vi "Obtain Request Events.vi"(8 "error in":errorcluster, 10 "Create New? (F)":bool) -> (0 "error out":errorcluster, 2 "UI Module Template Request Events":T1)   [LabVIEW 2024, in "UI Module Template.lvlib"]
doc: "This VI Obtains/Creates the Requests events that will be used for other modules to communicate with the module that owns this VI. These Requests events will be accessed only via Public API methods for this module.\n\n<b>NOTE</b>: The contents of this VI are automatically generated and modified by the <b>Tools > DQMH Consortium > DQMH</b> utilities. Consider using those utilities instead of making your own modifications to this VI.\n_____\nBased on DQMH Project Template 7.0.1.1316."
uses:
  UI Module Template.lvlib
  Request Events--cluster.ctl
  Stop Argument--cluster.ctl
  Show Panel Argument--cluster.ctl
  Hide Panel Argument--cluster.ctl
  Get Module Execution Status Argument--cluster.ctl
  Show Diagram Argument--cluster.ctl
  Get UI Reference Argument--cluster.ctl
  Get UI Reference (Reply Payload)--cluster.ctl
  Inserted Into Subpanel Argument--cluster.ctl
  Set Config (String) Argument--cluster.ctl
  Set Config Argument--cluster.ctl
  Config.ctl
  Get config Argument--cluster.ctl
  Get config (Reply Payload)--cluster.ctl
  Get Config (String) Argument--cluster.ctl
  Get Config (String) (Reply Payload)--cluster.ctl
  Generate Dummy Data Argument--cluster.ctl
panel:
  # "NOTE: The contents of this VI are automatically generated and modified by the Tools > DQMH Consortium > DQMH utilities. Consider using those utilities instead of making your own modifications to this VI."
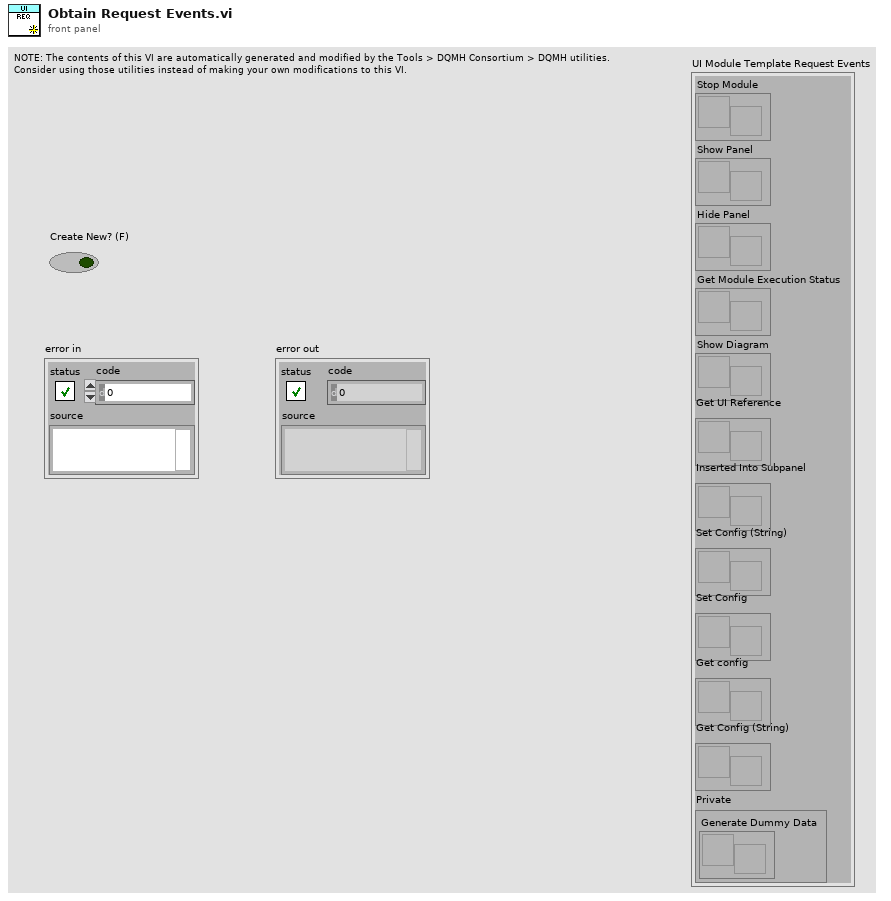
[diagram p1: front panel]
types:
  T1 = typedef "UI Module Template.lvlib/Request Events--cluster.ctl" = cluster{"Stop Module":refnum<user-event>, "Show Panel":refnum<user-event>, "Hide Panel":refnum<user-event>, "Get Module Execution Status":refnum<user-event>, "Show Diagram":refnum<user-event>, "Get UI Reference":refnum<user-event>, "Inserted Into Subpanel":refnum<user-event>, "Set Config (String)":refnum<user-event>, "Set Config":refnum<user-event>, "Get config":refnum<user-event>, "Get Config (String)":refnum<user-event>, "Private":cluster{"Generate Dummy Data":refnum<user-event>}}
  T2 = typedef "UI Module Template.lvlib/Generate Dummy Data Argument--cluster.ctl" = cluster{"Boolean":bool}
  T3 = typedef "UI Module Template.lvlib/Get Config (String) Argument--cluster.ctl" = cluster{"Wait Notifier":refnum<notifier>, "wait for reply":bool}
  T4 = typedef "UI Module Template.lvlib/Get config Argument--cluster.ctl" = cluster{"Wait Notifier":refnum<notifier>, "wait for reply":bool}
  T5 = typedef "UI Module Template.lvlib/Set Config Argument--cluster.ctl" = cluster{"Config":T6}
  T6 = typedef "UI Module Template.lvlib/Config.ctl" = cluster{"<ReplaceMe>":bool}
  T7 = typedef "UI Module Template.lvlib/Set Config (String) Argument--cluster.ctl" = cluster{"XML-String":string}
  T8 = typedef "UI Module Template.lvlib/Inserted Into Subpanel Argument--cluster.ctl" = cluster{"Boolean":bool}
  T9 = typedef "UI Module Template.lvlib/Get UI Reference Argument--cluster.ctl" = cluster{"Wait Notifier":refnum<notifier>, "wait for reply":bool}
  T10 = typedef "UI Module Template.lvlib/Hide Panel Argument--cluster.ctl" = cluster{"Hide Panel?":bool}
  T11 = typedef "UI Module Template.lvlib/Show Panel Argument--cluster.ctl" = cluster{"Show Panel?":bool}
  T12 = typedef "UI Module Template.lvlib/Show Diagram Argument--cluster.ctl" = cluster{"Debug?":bool}
  T13 = typedef "UI Module Template.lvlib/Get Module Execution Status Argument--cluster.ctl" = cluster{"Running?":bool}
  T14 = typedef "UI Module Template.lvlib/Stop Argument--cluster.ctl" = cluster{"Origin":string, "Exit via Stop Module Req?":bool, "Wait for Module to stop?":bool}
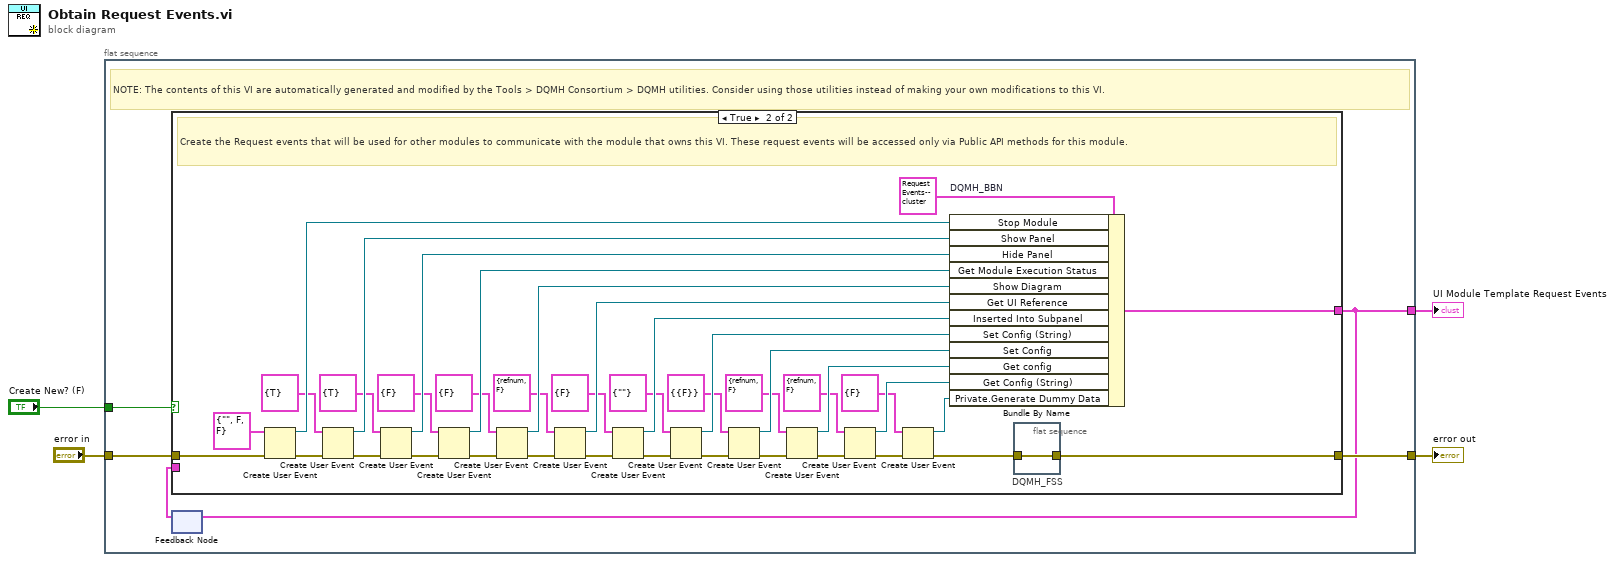
[diagram p0: block diagram]
diagram:
  n1 = flat-sequence {
    tunnel: [w9] -> w4
    tunnel: "error in" -> [w8]
    tunnel: [w6] -> w2
    tunnel: "Create New? (F)" -> [w5]
    frame #0 {
      # "NOTE: The contents of this VI are automatically generated and modified by the Tools > DQMH Consortium > DQMH utilities. Consider using those utilities instead of making your own modifications to this VI."
      n2 = feedback #1() -> (w7:T1)  [unwired: 1 in]
      n3 = case shown="True" w5 {
        tunnel: [w10 w41] -> w9
        tunnel: w8 -> [w10 w51]
        tunnel: [w11 w48] -> w6
        tunnel: w7 -> [w11 _]
        frame False {
          # "Obtain the Request events that were created in a previous call to this VI."
        }
        frame True {
          # "Create the Request events that will be used for other modules to communicate with the module that owns this VI. These request events will be accessed only via Public API methods for this module."
          n4 = Create User Event(user event datatype=T14 {"Origin"="", "Exit via Stop Module Req?"=FALSE, "Wait for Module to stop?"=FALSE} ("Stop Argument"), error in=w51) -> (user event=w49:refnum<user-event>, error out=w46:errorcluster)
          n5 = Create User Event(user event datatype=T11 {"Show Panel?"=TRUE} ("Show Panel Argument"), error in=w46) -> (user event=w45:refnum<user-event>, error out=w44:errorcluster)
          n6 = Create User Event(user event datatype=T10 {"Hide Panel?"=TRUE} ("Hide Panel Argument"), error in=w44) -> (user event=w43:refnum<user-event>, error out=w42:errorcluster)
          n7 = Create User Event(user event datatype=T13 {"Running?"=FALSE} ("Get Module Execution Status Argument"), error in=w42) -> (user event=w39:refnum<user-event>, error out=w40:errorcluster)
          n8 = Create User Event(user event datatype=T12 {"Debug?"=FALSE} ("Show Diagram Argument"), error in=w40) -> (user event=w36:refnum<user-event>, error out=w37:errorcluster)
          n9 = Create User Event(user event datatype=T9 {"Wait Notifier"=refnum, "wait for reply"=FALSE} ("Get UI Reference Argument"), error in=w37) -> (user event=w31:refnum<user-event>, error out=w32:errorcluster)
          n10 = Create User Event(user event datatype=T8 {"Boolean"=FALSE} ("Inserted Into Subpanel Argument"), error in=w32) -> (user event=w28:refnum<user-event>, error out=w29:errorcluster)
          n11 = Create User Event(user event datatype=T7 {"XML-String"=""} ("Set Config (String) Argument"), error in=w29) -> (user event=w25:refnum<user-event>, error out=w26:errorcluster)
          n12 = Create User Event(user event datatype=T5 {"Config"={"<ReplaceMe>"=FALSE}} ("Set Config Argument"), error in=w26) -> (user event=w22:refnum<user-event>, error out=w23:errorcluster)
          n13 = Create User Event(user event datatype=T4 {"Wait Notifier"=refnum, "wait for reply"=FALSE} ("Get config Argument"), error in=w23) -> (user event=w19:refnum<user-event>, error out=w20:errorcluster)
          n14 = Create User Event(user event datatype=T3 {"Wait Notifier"=refnum, "wait for reply"=FALSE} ("Get Config (String) Argument"), error in=w20) -> (user event=w16:refnum<user-event>, error out=w17:errorcluster)
          n15 = Create User Event(user event datatype=T2 {"Boolean"=FALSE} ("Generate Dummy Data Argument"), error in=w17) -> (user event=w13:refnum<user-event>, error out=w14:errorcluster)
          n16 = Bundle By Name "DQMH_BBN"(cluster=T1 {"Stop Module"=refnum, "Show Panel"=refnum, "Hide Panel"=refnum, "Get Module Execution Status"=refnum, "Show Diagram"=refnum, "Get UI Reference"=refnum, "Inserted Into Subpanel"=refnum, "Set Config (String)"=refnum, "Set Config"=refnum, "Get config"=refnum, "Get Config (String)"=refnum, "Private"={"Generate Dummy Data"=refnum}} ("output cluster"), "Stop Module"=w49, "Show Panel"=w45, "Hide Panel"=w43, "Get Module Execution Status"=w39, "Show Diagram"=w36, "Get UI Reference"=w31, "Inserted Into Subpanel"=w28, "Set Config (String)"=w25, "Set Config"=w22, "Get config"=w19, "Get Config (String)"=w16, "Private.Generate Dummy Data"=w13) -> (w48:T1)
          n17 = flat-sequence "DQMH_FSS" {
            tunnel: w14 -> [w52]
            tunnel: [w52] -> w41
            frame #0 {
            }
          }
        }
      }
      n18 = feedback-in #1(w6) -> ()
    }
  }
  "UI Module Template Request Events" <- w2
  "error out" <- w4
